vi "Query Limit Test Results.vi"(0 "VISA resource name":refnum<visa-resource-name>, 11 "error in (no error)":errorcluster) -> (4 "VISA resource name out":refnum<visa-resource-name>, 6 "Wide Limit Test Fail":bool, 8 "Narrow Limit Test Fail":bool, 15 "error out":errorcluster)   [LabVIEW 2021, in "Keithley 648X Series.lvlib"]
doc: "Queries the results of the latest limit test."
uses:
  <instrlib>/Keithley 648X Series/Keithley 648X Series.lvlib
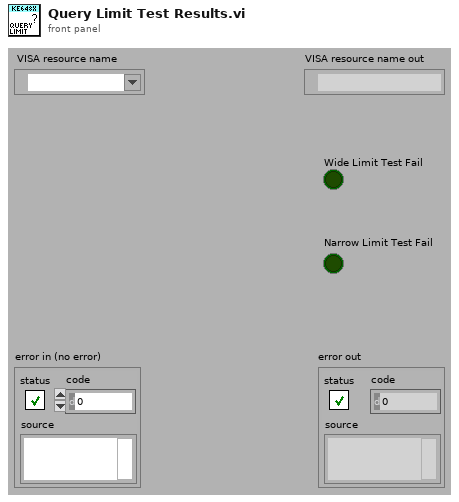
[diagram p1: front panel]
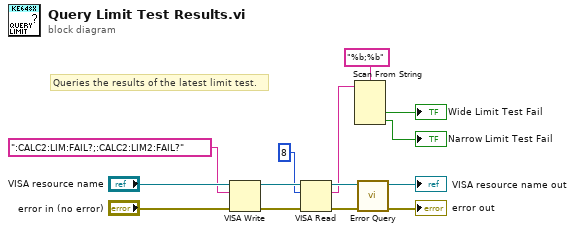
[diagram p0: block diagram]
diagram:
  # "Queries the results of the latest limit test."
  n1 = VISA Write(VISA resource name="VISA resource name", write buffer=":CALC2:LIM:FAIL?;:CALC2:LIM2:FAIL?", error in (no error)="error in (no error)") -> (VISA resource name out=w7:refnum<visa-resource-name>, error out=w6:errorcluster)  [unwired: 1 out]
  n2 = VISA Read(VISA resource name=w7, byte count=u32 8, error in (no error)=w6) -> (VISA resource name out=w8:refnum<visa-resource-name>, read buffer=w3:string, error out=w9:errorcluster)  [unwired: 1 out]
  n3 = Scan From String(format string="%b;%b", input string=w3) -> (output 1=→"Wide Limit Test Fail":bool, output 2=→"Narrow Limit Test Fail":bool)  [unwired: 4 in, 3 out]
  n4 = call <instrlib>:"Error Query.vi"("error in (no error)"=w9, "VISA resource name"=w8) -> ("error out"=→"error out":errorcluster, "VISA resource name out"=→"VISA resource name out":refnum<visa-resource-name>)  [unwired: 6 in, 2 out]
